vi "Sample Class Method API.vi"(8 "error in (no error)":errorcluster, 9 "String":string, 10 "Numeric":dbl, 11 "My Sample Class in":refnum<data-value>) -> (0 "error out":errorcluster, 2 "Boolean":bool, 3 "My Sample Class out":refnum<data-value>)   [LabVIEW 2016, in "My Sample Class.lvclass"]
uses:
  My Sample Class.lvclass
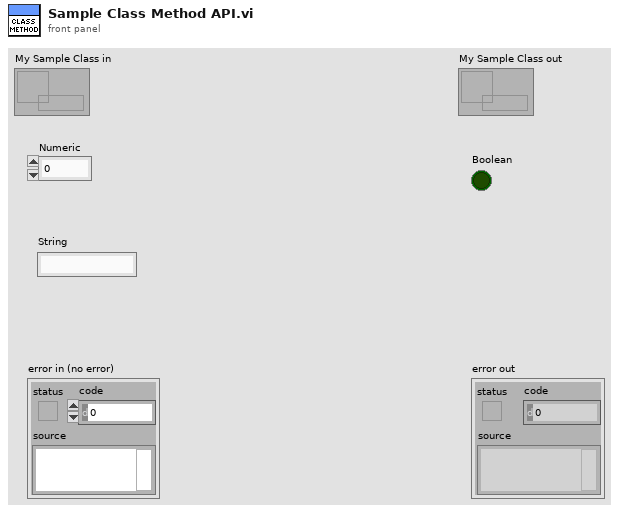
[diagram p1: front panel]
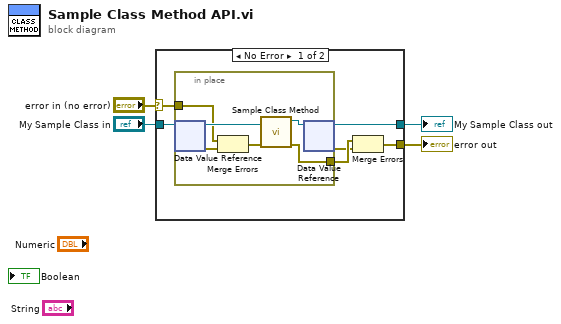
[diagram p0: block diagram]
diagram:
  n1 = case "Error Case Structure" shown="No Error" "error in (no error)" {
    selector: "error in (no error)" -> [w10 w17]
    tunnel: [w7 w17] -> w3
    tunnel: "My Sample Class in" -> [w6 _]
    tunnel: [w5 _] -> w1
    frame No Error {
      n2 = in-place {
        in-place-border: w10 -> [w14]
        in-place-border: [w13] -> w9
        n3 = in-place-dvr #1(w6) -> (w16:refnum<class "My Sample Class.lvclass">, w11:errorcluster)
        n4 = Merge Errors(w14, w11) -> (w12:errorcluster)
        n5 = call-dynamic "Sample Class Method.vi"(7:w16, "error in (no error)"=w12) -> ("error out"=w13:errorcluster, "My Sample Class out"=w15:refnum<class "My Sample Class.lvclass">)  [unwired: 7 in, 1 out]
        n6 = in-place-dvr #1(w15) -> (w5:refnum<data-value>, w8:errorcluster)
      }
      n7 = Merge Errors(w9, w8) -> (w7:errorcluster)
    }
    frame Error {
    }
  }
  "error out" <- w3
  "My Sample Class out" <- w1
